vi "Flush Text Log File.vi"(8 "error in (no error)":errorcluster, 11 "Text Log File in":refnum<class "Text Log File.lvclass">) -> (0 "error out":errorcluster, 3 "Text Log File out":refnum<class "Text Log File.lvclass">)   [LabVIEW 2012, in "Waveform Data Logger Engine.lvlib" / "Text Log File.lvclass"]
uses:
  Text Log File.lvclass
  Text Log File.lvclass/Text Log File.ctl
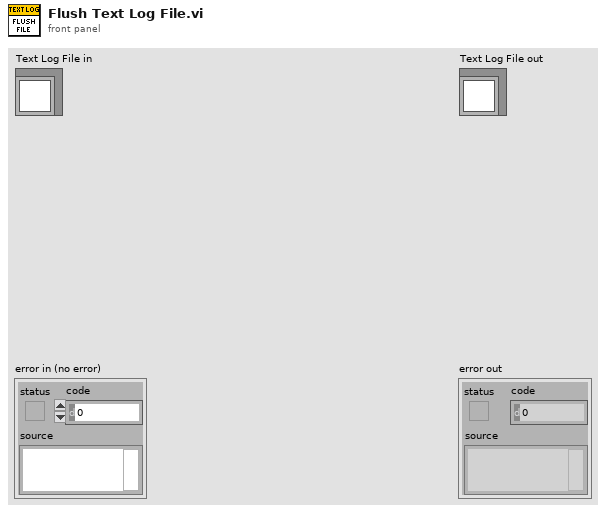
[diagram p1: front panel]
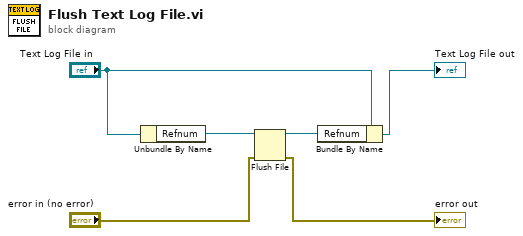
[diagram p0: block diagram]
diagram:
  n1 = Unbundle By Name("Text Log File in") -> ("Refnum"=w6:refnum<file>)
  n2 = Flush File(refnum=w6, error in="error in (no error)") -> (refnum out=w5:refnum<file>, error out=→"error out":errorcluster)
  n3 = Bundle By Name(cluster="Text Log File in", "Refnum"=w5) -> (→"Text Log File out":refnum<class "Text Log File.lvclass">)
